vi "Read_Key_IN.vi"(0 "VISA resource name":refnum<visa-resource-name> caption="VISA资源名称", 5 "错误输入（无错误）":errorcluster) -> (14 "VISA资源名称输出":refnum<visa-resource-name>, 15 "读取缓冲区":string, 16 "结果字符串":string, 17 "数组":string[](array[string]), 18 "Boolean array":bool[](array[boolean]), 19 "错误输出":errorcluster)   [LabVIEW 2018]
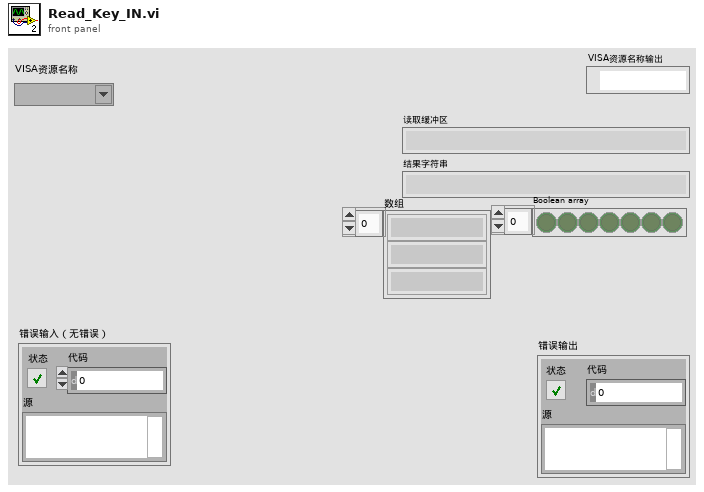
[diagram p1: front panel]
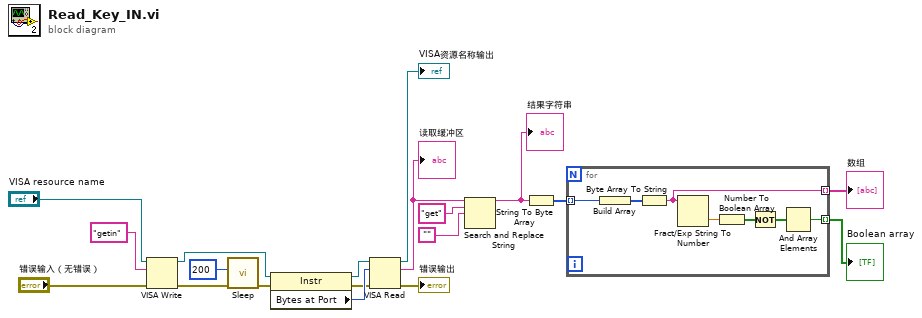
[diagram p0: block diagram]
diagram:
  n1 = VISA Write(VISA resource name="VISA resource name", write buffer="getin" ("写入缓冲区"), error in (no error)="错误输入（无错误）") -> (VISA resource name out=w15:refnum<visa-resource-name>, error out=w14:errorcluster)  [unwired: 1 out]
  n2 = call "Sleep.vi"("error in (no error)"=w14, "等待时间（毫秒）"=u32 200) -> ("error out"=w16:errorcluster)  [unwired: 9 in]
  n3 = property class="Instr"(reference=w15, error in=w16) -> (reference out=w17:refnum<visa-resource-name>, error out=w18:errorcluster, "Bytes at Port"=w19:u32)
  n4 = VISA Read(VISA resource name=w17, byte count=w19, error in (no error)=w18) -> (VISA resource name out=→"VISA资源名称输出":refnum<visa-resource-name>, read buffer=w11:string, error out=→"错误输出":errorcluster)  [unwired: 1 out]
  "读取缓冲区" <- w11
  n5 = Search and Replace String(input string=w11, search string="get" ("搜索字符串"), replace string="") -> (result string=w8:string)  [unwired: 5 in, 3 out]
  "结果字符串" <- w8
  n6 = String To Byte Array(string=w8) -> (unsigned byte array=w7:u8[])
  n7 = for {
    tunnel: w7 -> [w26] mode=indexing
    tunnel: [w24] -> w6 mode=indexing
    tunnel: [w20] -> w5 mode=indexing
    n8 = Build Array(w26) -> (w25:u8[])
    n9 = Byte Array To String(unsigned byte array=w25) -> (string=w24:string)
    n10 = Fract/Exp String To Number(string=w24) -> (number=w23:dbl)  [unwired: 3 in, 1 out]
    n11 = Number To Boolean Array(number=w23) -> (Boolean array=w22:bool[])
    n12 = Not(x=w22) -> (.not. x?=w21:bool[])
    n13 = And Array Elements(Boolean array=w21) -> (logical AND=w20:bool)
  }
  "数组" <- w6
  "Boolean array" <- w5
